vi "Heater Association (Set).vi"(6 "ISOBUS address":T2=-1 caption="ISOBUS address (-1)", 8 "error in":errorcluster, 10 "Heater UID":string, 11 "Mercury Reference In":T4) -> (0 "error out":errorcluster, 2 "Response":T1, 3 "Mercury Reference Out":T4, 4 "Valid?":T3)   [LabVIEW 2014, in "Mercury iXX.lvlib" / "Control Loop.lvlib"]
doc: "Set the UID of the associated heater to the control loop.\nSet value to 0 to unset association."
uses:
  Control Loop.lvlib
  Controls/Mercury Reference.ctl
  Controls/Comms Transport Layer.ctl
  Private/Controls/Query Dynamic Reference.ctl
  Controls/Is Valid LED.ctl
  Controls/ISOBus Address.ctl
  Controls/Response String.ctl
  Private/Controls/Command Verbs.ctl
  Mercury iXX.lvlib
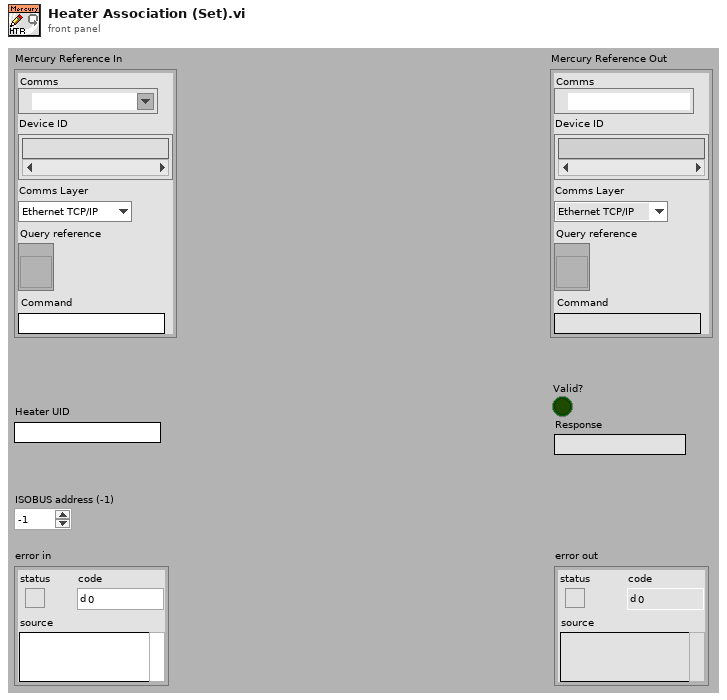
[diagram p1: front panel]
types:
  T1 = typedef "Mercury iXX.lvlib/Response String.ctl" = string
  T2 = typedef "Mercury iXX.lvlib/ISOBus Address.ctl" = i32
  T3 = typedef "Mercury iXX.lvlib/Is Valid LED.ctl" = bool
  T4 = typedef "Mercury iXX.lvlib/Mercury Reference.ctl" = cluster{"Comms":refnum<visa-resource-name>, "Device ID":string[], "Comms Layer":T5, "Command":string, "Query reference":T6}
  T5 = typedef "Mercury iXX.lvlib/Comms Transport Layer.ctl" = enum16{"Ethernet TCP/IP", "USB", "ISOBus - RS-232", "GPIB"}
  T6 = typedef "Mercury iXX.lvlib/Query Dynamic Reference.ctl" = refnum<vi>
  T7 = typedef "Mercury iXX.lvlib/Command Verbs.ctl" = string
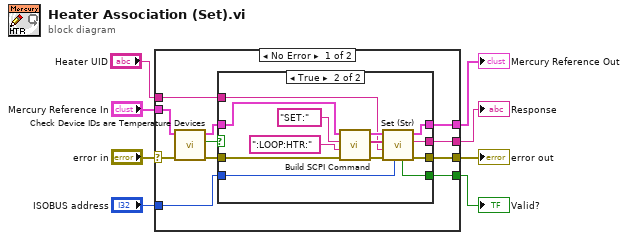
[diagram p0: block diagram]
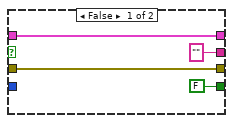
[diagram p2: hidden frame]
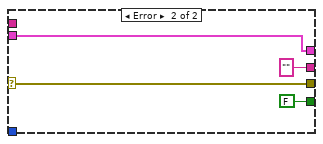
[diagram p3: hidden frame]
diagram:
  n1 = case shown="No Error" "error in" {
    selector: "error in" -> [w12 w40]
    tunnel: "Mercury Reference In" -> [w10 w37]
    tunnel: [w19 w37] -> w7
    tunnel: "ISOBUS address" -> [w18 _]
    tunnel: "Heater UID" -> [w17 _]
    tunnel: [w15 T1 "" ("Response")] -> w4
    tunnel: [w14 T3 FALSE ("Valid?")] -> w3
    tunnel: [w13 w40] -> w2
    frame No Error {
      n2 = call "Check Device IDs are Temperature Devices.vi"("error in"=w12, "Mercury Reference In"=w10) -> ("error out"=w11:errorcluster, "Valid?"=w16:bool, "Mercury Reference Out"=w9:T4)  [unwired: 7 out]
      n3 = case shown="True" w16 {
        tunnel: w9 -> [w22 w32]
        tunnel: [w22 w31] -> w19
        tunnel: w11 -> [w23 w25]
        tunnel: w18 -> [_ w24]
        tunnel: w17 -> [_ w26]
        tunnel: [T1 "" ("Response") w30] -> w15
        tunnel: [T3 FALSE ("Valid?") w29] -> w14
        tunnel: [w23 w28] -> w13
        frame False {
        }
        frame True {
          n4 = call "Build SCPI Command.vi"("error in"=w25, "Noun(s)"=":LOOP:HTR:" ("Command"), "Verb"=T7 "SET:", "Mercury Reference In"=w32) -> ("error out"=w36:errorcluster, "SCPI Message(s)"=w35:string[], "Mercury Reference Out"=w34:T4)  [unwired: 5 out]
          n5 = call "Set (Str).vi"("ISOBUS address"=w24, "error in"=w36, "Command Value (Str)"=w26, "SCPI Message(s)"=w35, "Mercury Reference In"=w34) -> ("error out"=w28:errorcluster, "Response"=w30:T1, "Mercury Reference Out"=w31:T4, "Valid?"=w29:T3)  [unwired: 3 out]
        }
      }
    }
    frame Error {
    }
  }
  "Mercury Reference Out" <- w7
  "error out" <- w2
  "Valid?" <- w3
  "Response" <- w4
